vi "Write From String Match.vi"(8 "error in (no error)":errorcluster, 10 "From String Match":string, 11 "Boolean in":refnum<class "Abs_Boolean.lvclass">) -> (0 "error out":errorcluster, 3 "Boolean out":refnum<class "Abs_Boolean.lvclass">)   [LabVIEW 2021, in "Abs_Boolean.lvclass"]
uses:
  Abs_Boolean.lvclass
  Abs_Boolean.lvclass/Abs_Boolean.ctl
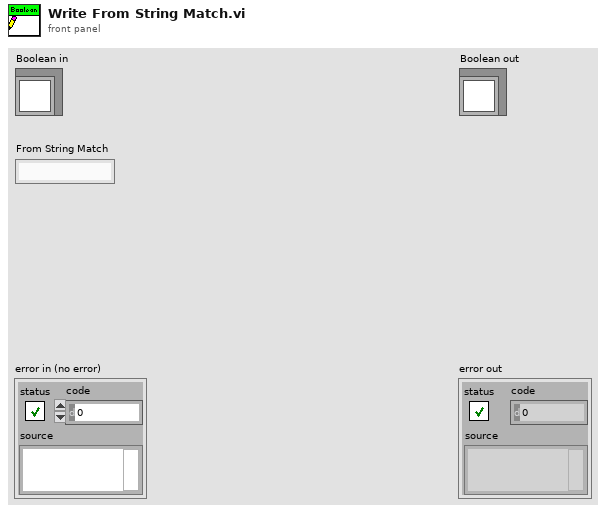
[diagram p1: front panel]
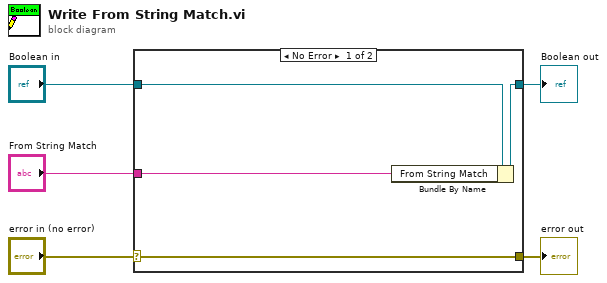
[diagram p0: block diagram]
diagram:
  n1 = case shown="No Error" "error in (no error)" {
    selector: "error in (no error)" -> [w9 w10]
    tunnel: [w9 w10] -> w4
    tunnel: [w7 w11] -> w2
    tunnel: "Boolean in" -> [w8 w11]
    tunnel: "From String Match" -> [w6 _]
    frame No Error {
      n2 = Bundle By Name(cluster=w8, "From String Match"=w6) -> (w7:refnum<class "Abs_Boolean.lvclass">)
    }
    frame Error {
    }
  }
  "error out" <- w4
  "Boolean out" <- w2
